vi "Analysis.Start End Interval, Generate DateTime Ranges.vi"(9 "Interval(Hrs)":dbl=24.0, 10 "EndTime":timestamp, 11 "StartTime":timestamp) -> (3 "DateRanges":cluster{"Start":timestamp, "End":timestamp}[](array[cluster]))   [LabVIEW 2024]
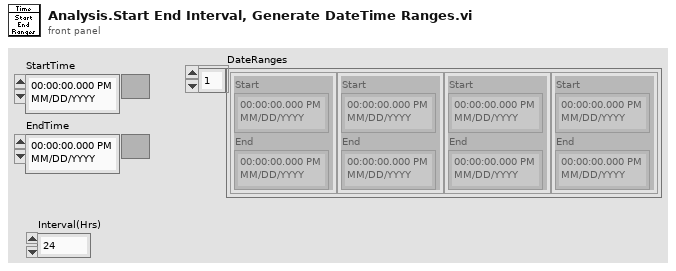
[diagram p1: front panel]
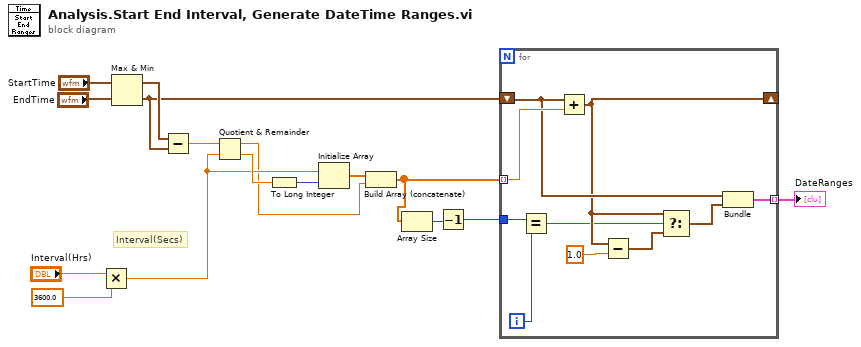
[diagram p0: block diagram]
diagram:
  # "Interval(Secs)"
  n1 = Multiply(x="Interval(Hrs)", y=3600.0) -> (x*y=w7:dbl)
  n2 = Max & Min(x="StartTime", y="EndTime") -> (max(x,y)=w14:timestamp, min(x,y)=w10:timestamp)
  n3 = Subtract(x=w14, y=w10) -> (x-y=w11:dbl)
  n4 = Quotient & Remainder(x=w11, y=w7) -> (x-y*floor(x/y)=w5:dbl, floor(x/y)=w8:dbl)
  n5 = To Long Integer(number=w8) -> (32bit integer=w9:i32)
  n6 = Initialize Array(w7, w9) -> (w6:dbl[])
  n7 = Build Array (concatenate)(w6, w5) -> (w4:dbl[])
  n8 = Array Size(array=w4) -> (size(s)=w3:i32)
  n9 = Decrement(x=w3) -> (x-1=w2:i32)
  n10 = for {
    tunnel: w4 -> [w26] mode=indexing
    shift-right: [w19] -> _
    shift-left: w10 -> [w24]
    tunnel: [w23] -> w1 mode=indexing
    tunnel: w2 -> [w22]
    i -> [w21]
    n11 = Equal?(x=w22, y=w21) -> (x = y?=w17:bool)
    n12 = Add(x=w24, y=w26) -> (x+y=w19:timestamp)
    n13 = Subtract(x=w19, y=1.0) -> (x-y=w20:timestamp)
    n14 = Select(t=w19, s=w17, f=w20) -> (s? t:f=w18:timestamp)
    n15 = Bundle(w24, w18) -> (w23:cluster{timestamp, timestamp})  [unwired: 1 in]
  }
  "DateRanges" <- w1
